vi "Write Exception Status.vi"(8 "error in (no error)":errorcluster, 10 "exception status":u8 format="%02x", 11 "device data model in":refnum<class "Standard Data Model.lvclass">) -> (0 "error out":errorcluster, 3 "device data model out":refnum<class "Standard Data Model.lvclass">)   [LabVIEW 2020, in "SubVIs.lvlib" / "Standard Data Model.lvclass"]
doc: "Sets the exception status in the device data model."
uses:
  <vilib>/Modbus/subvis/Data and Functions/Standard Data Model/Standard Data Model.lvclass
  <vilib>/Modbus/subvis/Data and Functions/Standard Data Model/Standard Data Model.lvclass/Standard Data Model.ctl
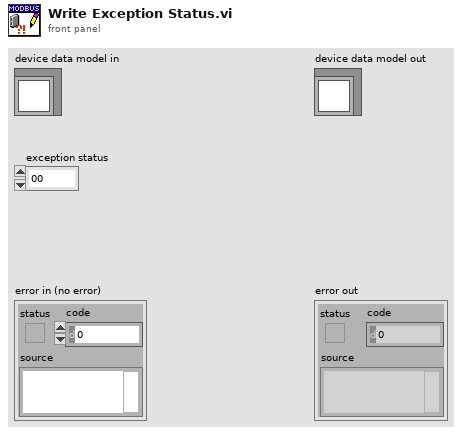
[diagram p1: front panel]
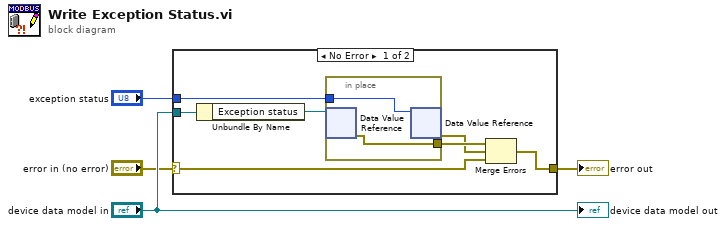
[diagram p0: block diagram]
diagram:
  n1 = case shown="No Error" "error in (no error)" {
    selector: "error in (no error)" -> [w6 w14]
    tunnel: [w11 w14] -> w4
    tunnel: "device data model in" -> [w10 _]
    tunnel: "exception status" -> [w8 _]
    frame No Error {
      n2 = Unbundle By Name(w10) -> ("Exception status"=w9:refnum<data-value>)
      n3 = in-place {
        in-place-border: w8 -> [w13]
        in-place-border: [w12] -> w7
        n4 = in-place-dvr #1(w9) -> (w12:errorcluster)  [unwired: 1 out]
        n5 = in-place-dvr #1(w13) -> (w5:errorcluster)  [unwired: 1 out]
      }
      n6 = Merge Errors(w7, w5, w6) -> (w11:errorcluster)
    }
    frame Error {
    }
  }
  "error out" <- w4
  "device data model out" <- "device data model in"
